vi "PLC.Debug.CheckStatus.vi"(8 "error in (no error)":errorcluster, 10 "PLCcheckstatus":T1, 11 "Idx":i32) -> (0 "error out":errorcluster, 2 "PCcheckstatus":T2)   [LabVIEW 2016]
doc: "Connect to PLC\n\nWabco 2017 All right reserved\nAuthor: maciej.szupienko@wabco-auto.com"
uses:
  LowLevel/PLC.DataBlock.PCcheckstatus.ctl
  LowLevel/PLC.DataBlock.PLCcheckstatus.ctl
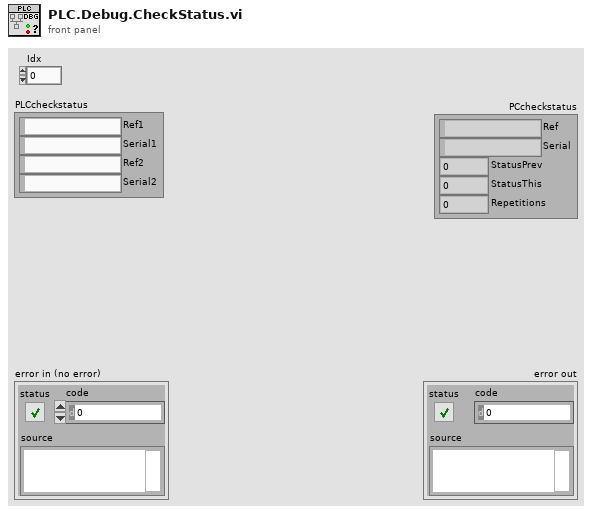
[diagram p1: front panel]
types:
  T1 = typedef "PLC.DataBlock.PLCcheckstatus.ctl" = cluster{"Ref1":string, "Serial1":string, "Ref2":string, "Serial2":string}
  T2 = typedef "PLC.DataBlock.PCcheckstatus.ctl" = cluster{"Ref":string, "Serial":string, "StatusPrev":i8, "StatusThis":i8, "Repetitions":u8}
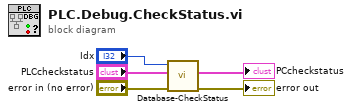
[diagram p0: block diagram]
diagram:
  n1 = call "Database-CheckStatus.vi"("error in"="error in (no error)", "PLCcheckstatus"="PLCcheckstatus", "Idx"="Idx") -> ("error out"=→"error out":errorcluster, "PCcheckstatus"=→"PCcheckstatus":T2)  [unwired: 7 in]
